vi "Simple Add.vi"() -> ()   [LabVIEW 2018]
panel:
  out "Boolean":bool
  out "x+y":dbl
  in  "y":dbl
  in  "x":dbl
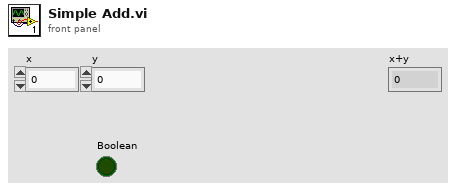
[diagram p1: front panel]
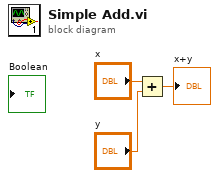
[diagram p0: block diagram]
diagram:
  n1 = Add(x="x", y="y") -> (x+y=→"x+y":dbl)
